vi "Set by Name.vi"(8 "error in":errorcluster, 9 "Value":bool, 10 "Channel Name":string, 11 "DIG_IO in":refnum<class "DIG_IO.lvclass">) -> (0 "error out":errorcluster, 3 "DIG_IO out":refnum<class "DIG_IO.lvclass">)   [LabVIEW 2019, in "DIG_IO.lvlib" / "DIG_IO.lvclass"]
uses:
  Library/DIG_IO.lvclass
  C:/Users/Public/Documents/Development/builds/Instruments/Instruments.lvlibp/Library/Instruments.lvclass
  Library/DIG_IO.lvclass/DIG_IO.ctl
  builds/Instruments/Instruments.lvlibp/Private/Polymorphic/Special/Event from Boolean.vi
  builds/Instruments/Instruments.lvlibp/Accessors/Command with Logging.vi
  builds/Instruments/Instruments.lvlibp/Library/Instruments.lvclass
  builds/Instruments/Instruments.lvlibp
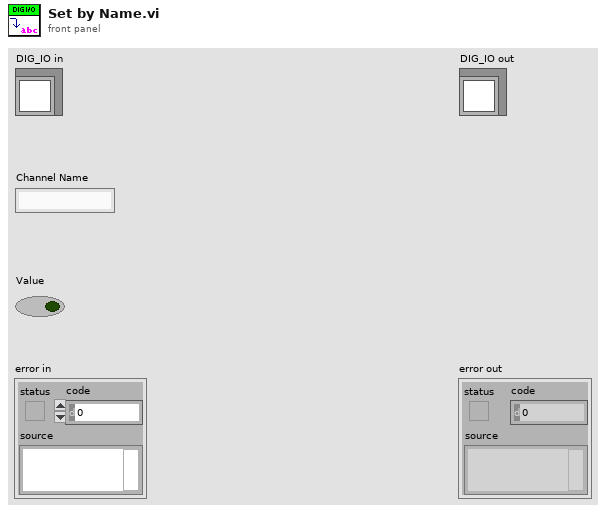
[diagram p1: front panel]
types:
  T1 = cluster{"Timestamp":timestamp, "Description":string, "Data":string}
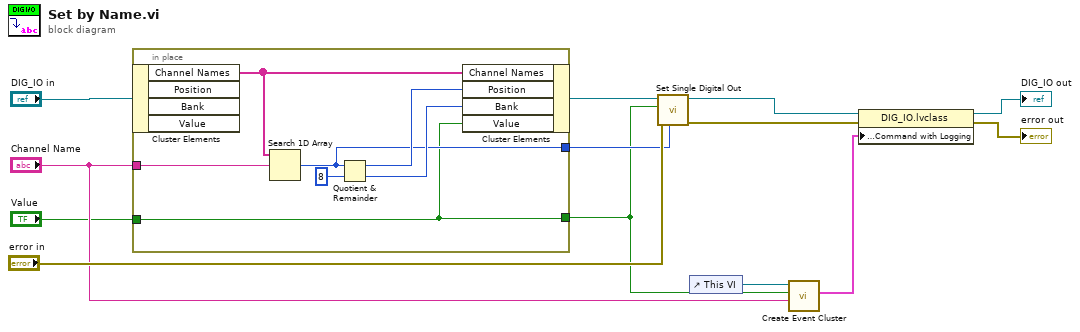
[diagram p0: block diagram]
diagram:
  n1 = in-place {
    in-place-border: "Channel Name" -> [w19]
    in-place-border: "Value" -> [w14]
    in-place-border: [w15] -> w3
    in-place-border: [w14] -> w1
    n2 = in-place-cluster #1("DIG_IO in") -> ("Channel Names"=w20:string[])  [unwired: 3 out]
    n3 = Search 1D Array(1D array=w20, element=w19) -> (index of element=w15:i32)  [unwired: 1 in]
    n4 = Quotient & Remainder(x=w15, y=8) -> (x-y*floor(x/y)=w17:i32, floor(x/y)=w16:i32)
    n5 = in-place-cluster #1("Channel Names"=w20, "Position"=w17, "Bank"=w16, "Value"=w14) -> (w2:refnum<class "DIG_IO.lvclass">)
  }
  n6 = call "Set Single Digital Out.vi"("Target Digital out"=w3, "error in"="error in", "Value to Write"=w1, "DIG_IO in"=w2) -> ("error out"=w11:errorcluster, "DIG_IO out"=w13:refnum<class "DIG_IO.lvclass">)  [unwired: 6 in]
  n7 = control-ref of="This VI"() -> (w8:refnum<vi>)
  n8 = call-poly "Create Event Cluster.vi"("Name"="Channel Name", "Value"=w1, "VI Refnum"=w8) -> ("Event Data"=w7:T1)  [unwired: 8 in]
  n9 = property class="DIG_IO.lvclass"(reference=w13, error in=w11, "Accessors:Logging:Command with Logging"=w7) -> (reference out=→"DIG_IO out":refnum<class "DIG_IO.lvclass">, error out=→"error out":errorcluster)
